vi "Locked columns Write.vi"(4 "error in (no error)":errorcluster, 5 "Value":i32[](array[numeric]), 6 "Container State":T6, 7 "Display State In":T1) -> (0 "error out":errorcluster, 3 "Display State Out":T1)   [LabVIEW 2015, in "KTable.xctl"]
uses:
  KTable.xctl
  <vilib>/_xctls/Container State.ctl
  State.ctl
  ColumnSpec.ctl
  ColumnType.ctl
  Table Properties.ctl
  Events.ctl
  Event Data.ctl
  Event Type.ctl
  <vilib>/_xctls/XControlSupport.lvlib
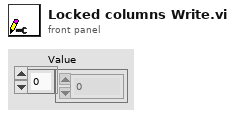
[diagram p1: front panel]
types:
  T1 = typedef "KTable.xctl/State.ctl" = cluster{"Columns":T2[], "Listbox":refnum<vi>, "Default row":string[], "Properties":T4, "Events":T5, "Locked":bool[][], "Size":cluster{"Rows":i32, "Columns":i32}, "rings":i32[][], "DefColors":u32[]}
  T2 = typedef "KTable.xctl/ColumnSpec.ctl" = cluster{"Name":string, "Type":T3, "Width":i32, "Strings":string[], "Position":enum16{"Left", "Center", "Right"}, "locked":bool, "cds":cluster{"Strings":string[]}[][]}
  T3 = typedef "KTable.xctl/ColumnType.ctl" = enum16{"String", "Enum", "Int", "Double", "Boolean", "Ring", "Formula", "Color"}
  T4 = typedef "KTable.xctl/Table Properties.ctl" = cluster{"Vertical scrollbar":bool, "User add/delete":bool, "Max rows":i32, "Row headers":bool}
  T5 = typedef "KTable.xctl/Events.ctl" = cluster{"Items Changed":refnum<user-event>}
  T6 = typedef "XControlSupport.lvlib/Container State.ctl" = cluster{"Indicator?":bool, "Run Mode?":bool, " Refnum":refnum<vi>}
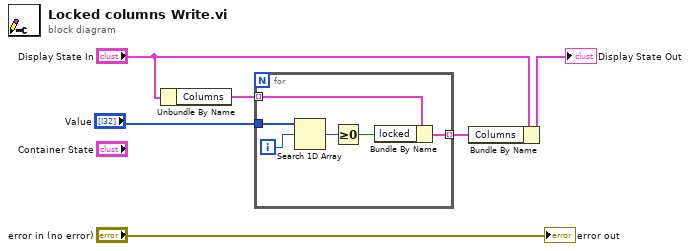
[diagram p0: block diagram]
diagram:
  n1 = Unbundle By Name("Display State In") -> ("Columns"=w3:T2[])
  n2 = for {
    tunnel: w3 -> [w12] mode=indexing
    tunnel: [w11] -> w2 mode=indexing
    tunnel: "Value" -> [w10]
    i -> [w9]
    n3 = Search 1D Array(1D array=w10, element=w9) -> (index of element=w8:i32)  [unwired: 1 in]
    n4 = Greater Or Equal To 0?(x=w8) -> (x >= 0?=w7:bool)
    n5 = Bundle By Name(cluster=w12, "locked"=w7) -> (w11:T2)
  }
  n6 = Bundle By Name(cluster="Display State In", "Columns"=w2) -> (→"Display State Out":T1)
  "error out" <- "error in (no error)"
